vi "GlobalUserBin.vi"() -> ()   [LabVIEW 2010]
panel:
  out "User Bin":bool
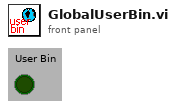
[diagram p1: front panel]
diagram:
